vi "Test Batch Run with Broken Tests.vi"(8 "error in (no error)":errorcluster) -> (0 "error out":errorcluster)   [LabVIEW 2013]
uses:
  classes/Test/Test.lvclass
  classes/Test Runner/Test Runner.lvclass
  classes/Assert/Assert.lvclass
  test-runner/test-brokenTests/Test Runner.BrokenTest.lvclass
panel:
  out "Test VIs":path[](array[path])
  out "error out 2":errorcluster
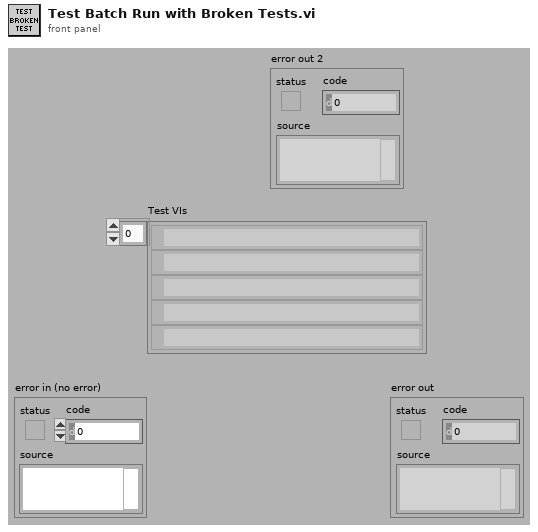
[diagram p1: front panel]
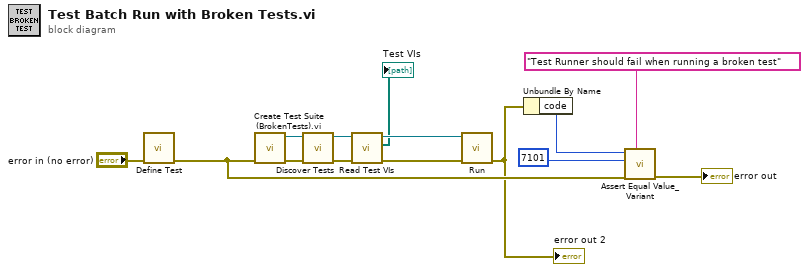
[diagram p0: block diagram]
diagram:
  n1 = call "Define Test.vi"("error in (no error)"="error in (no error)") -> ("error out"=w4:errorcluster)  [unwired: 10 in]
  n2 = call "Create Test Suite (BrokenTests).vi.vi"("error in (no error)"=w4) -> ("error out"=w10:errorcluster, "Test Runner.BrokenTests"=w11:refnum<class "Test Runner.BrokenTest.lvclass">)  [unwired: 9 in]
  n3 = call "Discover Tests.vi"("error in (no error)"=w10, "Test Runner in"=w11) -> ("error out"=w7:errorcluster, "Test Runner out"=w9:refnum<class "Test Runner.BrokenTest.lvclass">)  [unwired: 8 in]
  n4 = call "Read Test VIs.vi"("error in (no error)"=w7, "Test Runner in"=w9) -> ("error out"=w6:errorcluster, "Test VIs"=→"Test VIs":path[], "Test Runner out"=w8:refnum<class "Test Runner.BrokenTest.lvclass">)  [unwired: 7 in]
  n5 = call "Run.vi"("error in (no error)"=w6, "Test Runner in"=w8) -> ("error out"=w3:errorcluster)  [unwired: 8 in, 1 out]
  "error out 2" <- w3
  n6 = Unbundle By Name(w3) -> ("code"=w2:i32)
  n7 = call "Assert Equal Value_Variant.vi"("Label"="Test Runner should fail when running a broken test", "error in (no error)"=w4, "Y"=7101 ("code"), "X"=w2) -> ("error out"=→"error out":errorcluster)  [unwired: 7 in]
